vi "Read Headers.vi"(8 "error in (no error)":errorcluster, 11 "XML in":refnum<class "XML.lvclass">) -> (0 "error out":errorcluster, 1 "Header Values":string[](array[string]), 2 "Header Names":string[](array[string]), 3 "XML out":refnum<class "XML.lvclass">)   [LabVIEW 2017, in "XML.lvlib" / "XML.lvclass"]
uses:
  <vilib>/gpm_packages/@cs/persistence/source/XML/XML.lvclass
  <vilib>/gpm_packages/@cs/persistence/source/XML/XML.lvclass/XML.ctl
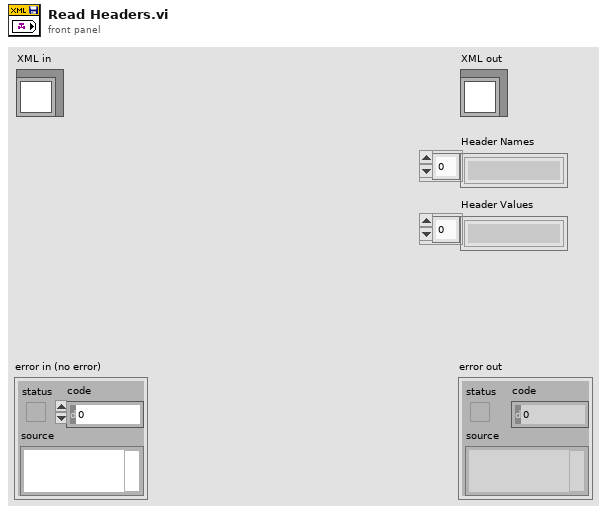
[diagram p1: front panel]
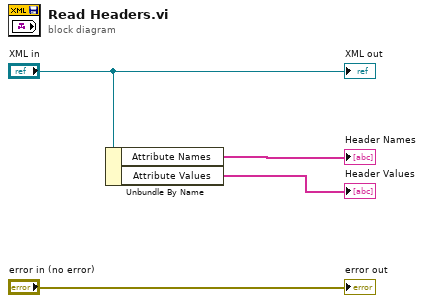
[diagram p0: block diagram]
diagram:
  n1 = Unbundle By Name("XML in") -> ("Attribute Names"=→"Header Names":string[], "Attribute Values"=→"Header Values":string[])
  "error out" <- "error in (no error)"
  "XML out" <- "XML in"
